vi "SetIntFeatureValue.vi"(8 "intValue":i32, 9 "pFeatureName":string, 10 "handle":i64, 11 "error in (no error)":errorcluster) -> (3 "error out":errorcluster)   [LabVIEW 2016]
uses:
  MVSDKmd.dll
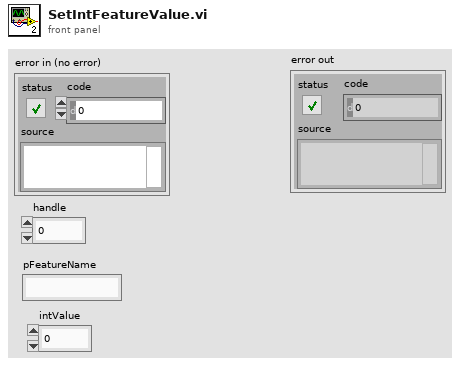
[diagram p1: front panel]
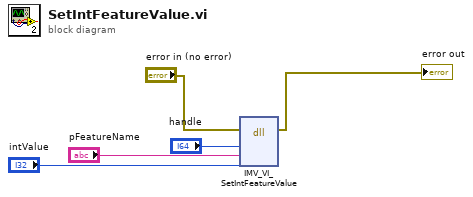
[diagram p0: block diagram]
diagram:
  n1 = dll-call lib="MVSDKmd.dll" fn="IMV_VI_SetIntFeatureValue"(error in="error in (no error)", "handle"="handle", "pFeatureName"="pFeatureName", "intValue"="intValue") -> (error out=→"error out":errorcluster)  [unwired: 6 in, 1 out]
